vi "Cleanup Block Diagram.vi"(8 "error in (no error)":errorcluster, 10 "Clean Up Options":T1={"Alignment"=enum."Gravity", "Rules"=enum."Strict", "Max Heuristic Iterations"=20, "Max Simplex Iterations"=20, "Block Padding"={"Horizontal"=50, "Vertical"=30}, "Wire Padding"={"Horizontal"=7, "Vertical"=5}, "Auto-Tune by Topology"=FALSE, "Fine-Tune Y Positions"=FALSE, "Align All Controls on Left"=TRUE, "Align All Indicators on Right"=TRUE, "Use Array Dimension Heuristics"=FALSE}, 11 "VI Path":path) -> (0 "error out":errorcluster, 3 "VI Path Out":path)   [LabVIEW 2016, in "SLL Class DVR API Generator.lvlib"]
uses:
  SLL Class DVR API Generator.lvlib
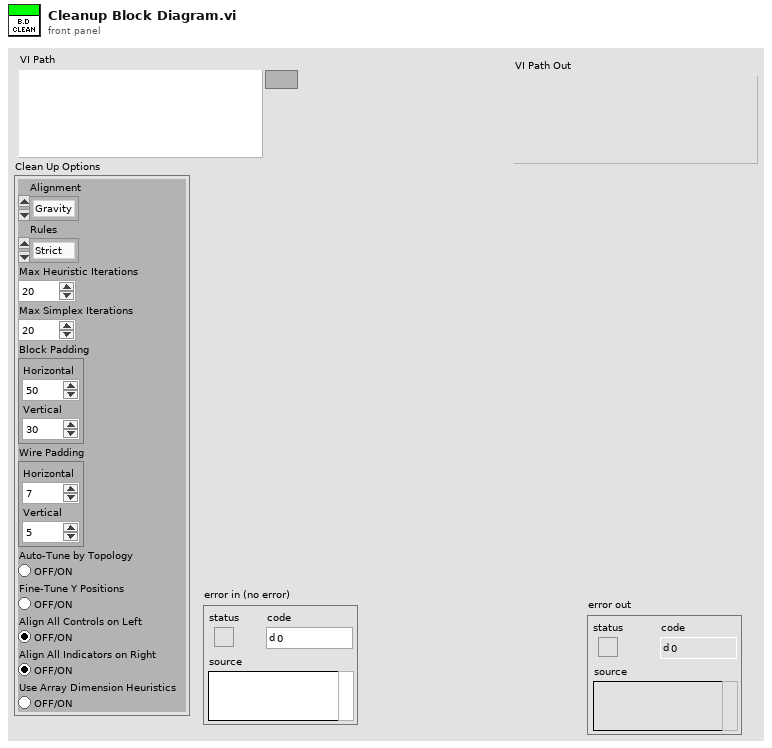
[diagram p1: front panel]
types:
  T1 = cluster{"Alignment":enum32{"Left", "Right", "Hybrid", "Center", "Gravity"}, "Rules":enum32{"Strict", "Allow Wires Under Labels", "Allow Wires Under Lead Nodes", "Allow Wires Under Wide Blocks"}, "Max Heuristic Iterations":u32, "Max Simplex Iterations":u32, "Block Padding":cluster{"Horizontal":i32, "Vertical":i32}, "Wire Padding":cluster{"Horizontal":i32, "Vertical":i32}, "Auto-Tune by Topology":bool, "Fine-Tune Y Positions":bool, "Align All Controls on Left":bool, "Align All Indicators on Right":bool, "Use Array Dimension Heuristics":bool}
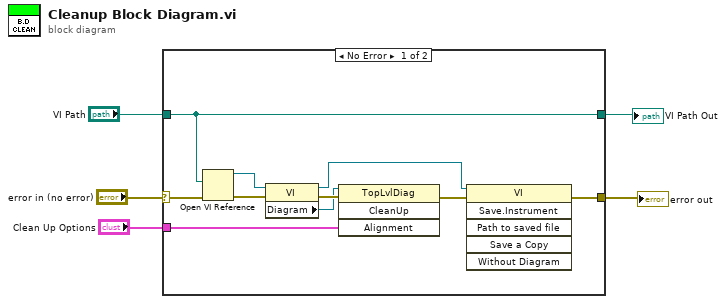
[diagram p0: block diagram]
diagram:
  n1 = case shown="No Error" "error in (no error)" {
    selector: "error in (no error)" -> [w15 w17]
    tunnel: [w8 w17] -> w4
    tunnel: "VI Path" -> [w12 w16]
    tunnel: [w12 w16] -> w2
    tunnel: "Clean Up Options" -> [w6 _]
    frame No Error {
      n2 = Open VI Reference(vi path=w12, error in (no error)=w15) -> (vi reference=w13:refnum<vi>, error out=w14:errorcluster)  [unwired: 4 in]
      n3 = property class="VI"(reference=w13, error in=w14) -> (reference out=w7:refnum<vi>, error out=w10:errorcluster, "Diagram"=w9:refnum<vi>)
      n4 = invoke class="TopLvlDiag" method="CleanUp"(reference=w9, error in=w10, "Alignment"=w6) -> (error out=w11:errorcluster)  [unwired: 1 in, 3 out]
      n5 = invoke class="VI" method="Save.Instrument"(reference=w7, error in=w11) -> (error out=w8:errorcluster)  [unwired: 4 in, 5 out]
    }
    frame Error {
    }
  }
  "error out" <- w4
  "VI Path Out" <- w2
